vi "StateDiagramGraph_Create.vi"(0 "reference":refnum<class "StateDiagramGraph.lvclass">, 1 "StateDiagramData":T1={"VI-Path"=path "", "ShowOption"=enum."Show Relative Path"}, 5 "error in (no error)":errorcluster) -> (14 "reference out":refnum<class "StateDiagramGraph.lvclass">, 19 "error out":errorcluster)   [LabVIEW 2014, in "StateDiagramGraph.lvclass"]
doc: "Creates and initializes a new StateDiagramGraph object.\n\nThis object should be destroyed using a StateDiagramGraph destructor VI or a virtual base class destructor VI.\n\n[GOOP 2.1]"
uses:
  <resource>/Framework/Providers/Open_GDS/UML/StateDiagramGraph_class/StateDiagramGraph.lvclass
  <resource>/Framework/Providers/Open_GDS/UML/StateDiagramGraph_class/private/StateDiagramData.ctl
  <resource>/Framework/Providers/Open_GDS/UML/StateDiagramGraph_class/private/ViPathShowOption.ctl
  <resource>/Framework/Providers/Open_GDS/UML/Graph_class/Graph.lvclass
panel:
  # "The input reference should only\nbe wired when this method is called\nby a sub class constructor."
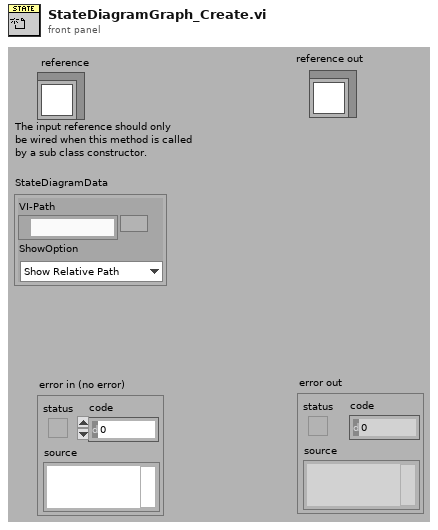
[diagram p1: front panel]
types:
  T1 = typedef "StateDiagramGraph.lvclass/StateDiagramData.ctl" = cluster{"VI-Path":path, "ShowOption":T2}
  T2 = typedef "StateDiagramGraph.lvclass/ViPathShowOption.ctl" = enum16{"Don't Show", "Show Relative Path", "Show Absolute Path"}
  T3 = typedef "StateDiagramGraph.lvclass/ObjectAttributes.ctl" = cluster{"StateDiagramData":T1}
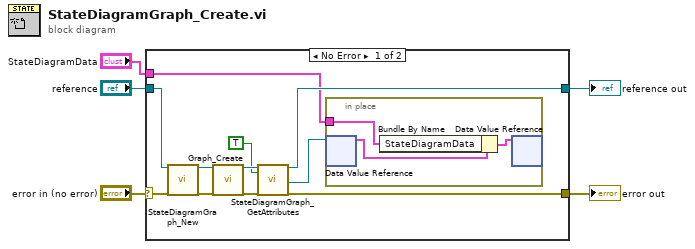
[diagram p0: block diagram]
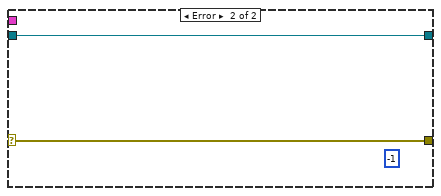
[diagram p2: hidden frame]
diagram:
  n1 = case shown="No Error" "error in (no error)" {
    selector: "error in (no error)" -> [w16 w21]
    tunnel: [w11 w20] -> w5
    tunnel: [w9 w21] -> w4
    tunnel: "reference" -> [w15 w20]
    tunnel: "StateDiagramData" -> [w6 _]
    frame No Error {
      n2 = call <resource>:"StateDiagramGraph_New.vi"("reference in"=w15, "error in (no error)"=w16) -> ("reference out"=w14:refnum<class "StateDiagramGraph.lvclass">, "error out"=w13:errorcluster)  [unwired: 2 in, 14 out]
      n3 = call <resource>:"Graph_Create.vi"("reference"=w14, "error in (no error)"=w13) -> ("reference out"=w12:refnum<class "StateDiagramGraph.lvclass">, "error out"=w10:errorcluster)  [unwired: 1 in, 15 out]
      n4 = call <resource>:"StateDiagramGraph_GetAttributes.vi"("reference in"=w12, "OnlyGetDvrReference(False)"=TRUE, "error in (no error)"=w10) -> ("reference out"=w11:refnum<class "StateDiagramGraph.lvclass">, "DataRef"=w7:refnum<data-value>, "error out"=w9:errorcluster)  [unwired: 13 in, 1 out]
      n5 = in-place {
        in-place-border: w6 -> [w18]
        n6 = in-place-dvr #1(w7) -> (w19:T3)  [unwired: 1 out]
        n7 = Bundle By Name(cluster=w19, "StateDiagramData"=w18) -> (w17:T3)
        n8 = in-place-dvr #1(w17) -> ()  [unwired: 2 out]
      }
    }
    frame Error {
      (unwired) -1 ("Nr of open handles")
    }
  }
  "error out" <- w4
  "reference out" <- w5
